vi "Begin.vi"(8 "error in":errorcluster) -> (0 "error out":errorcluster)   [LabVIEW 2014]
doc: "Called before other user functions, this VI is expected to open initial I/O refnums, load in file data, and do all program initialization. Notice that the <B>error out</B> terminal is simply used for data flow. Wiring it to other structures or subVIs ensures that this VI runs first."
uses:
  <vilib>/Rock Robotics/WPI/SafetyOutput/WPI_SafetyOutputConfigMenu.ctl
  <vilib>/Rock Robotics/WPI/DriverStation/WPI_DriverStationRobotMode2.ctl
  <vilib>/Rock Robotics/WPI/Joystick/WPI_JoystickDeviceEnum.ctl
  <vilib>/Rock Robotics/SystemInterfaces/DIO/FPGA_DIOPWMChannel.ctl
  Robot Global Data.vi
  <vilib>/Rock Robotics/Network Tables/SD Write String Array.vi
  <vilib>/Rock Robotics/WPI/RobotDrive/WPI_RobotDriveOpen4MotorWithJaguar.vi
panel:
  in  "error in 2":errorcluster
  out "error out 2":errorcluster
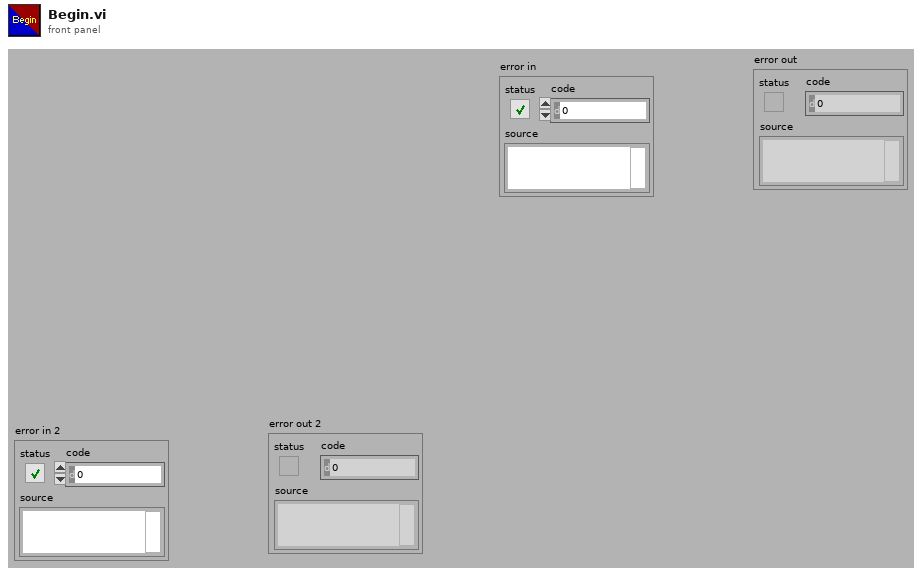
[diagram p1: front panel]
types:
  T1 = typedef "FPGA_DIOPWMChannel.ctl" = enum8{"PWM 0", "PWM 1", "PWM 2", "PWM 3", "PWM 4", "PWM 5", "PWM 6", "PWM 7", "PWM 8", "PWM 9", "PWM MXP 0", "PWM MXP 1", "PWM MXP 2", "PWM MXP 3", "PWM MXP 4", "PWM MXP 5", "PWM MXP 6", "PWM MXP 7", "PWM MXP 8", "PWM MXP 9", "Invalid"}
  T2 = typedef "WPI_JoystickDeviceEnum.ctl" = enum16{"USB 0", "USB 1", "USB 2", "USB 3", "USB 4", "USB 5"}
  T3 = typedef "WPI_DriverStationRobotMode2.ctl" = enum16{"Autonomous Disabled", "Autonomous Enabled", "Teleop Disabled", "Teleop Enabled", "Disconnected", "Finish", "Test Disabled", "Test Enabled", "Emergency Stopped"}
  T4 = typedef "WPI_SafetyOutputConfigMenu.ctl" = enum16{"Enable", "Disable"}
  T5 = typedef "WPI_JoystickDevRef.ctl" = cluster{"Device":T2}
  T6 = typedef "WPI_RobotDriveDevRef.ctl" = cluster{"DevStatus":errorcluster, "Motors[]":T7[], "Square Inputs":bool, "Max Output":dbl}
  T7 = typedef "WPI_MotorControlDeviceRef.ctl" = cluster{"DeviceStatus":errorcluster, "Type":T8, "PWM":cluster{"Controller":T9, "PWM Channel":T1, "DeadBand":T10}, "CAN":cluster{"Device Number":u8, "Control Mode":T11, "Semaphore":T12, "Max Vout":dbl, "TalonSRX Control Mode":T13}, "Invert":bool, "TransformRef":T14, "InvTransformRef":T14}
  T8 = typedef "WPI_MotorControlType.ctl" = enum16{"PWM", "CAN", "CANTalonSRX"}
  T9 = typedef "FPGA_TypedefDigitalModule.ctl" = enum16{"Controller 1"}
  T10 = typedef "WPI_PWMDeadband.ctl" = cluster{"Name":string, "maxPositivePwm":i32, "minPositivePwm":i32, "centerPwm":i32, "maxNegativePwm":i32, "minNegativePwm":i32, "angularRange":u16}
  T11 = typedef "WPI_CANJaguar_ControlMode.ctl" = enum8{"Percent VBus", "Current", "Speed", "Position", "Voltage"}
  T12 = typedef "Semaphore RefNum" = refnum<k1>
  T13 = typedef "WPI_CANTalonSRX_APIControlMode.ctl" = enum8{"Percent VBus", "Speed", "Position", "Slave", "Unchanged / Invalid"}
  T14 = typedef "WPI_PWMTransform_ConPane.ctl" = refnum<vi>
  T15 = typedef "WPI_ServoDeviceRef.ctl" = cluster{"DeviceStatus":errorcluster, "Controller":T9, "PWM Channel":T1, "DeadBand":T10}
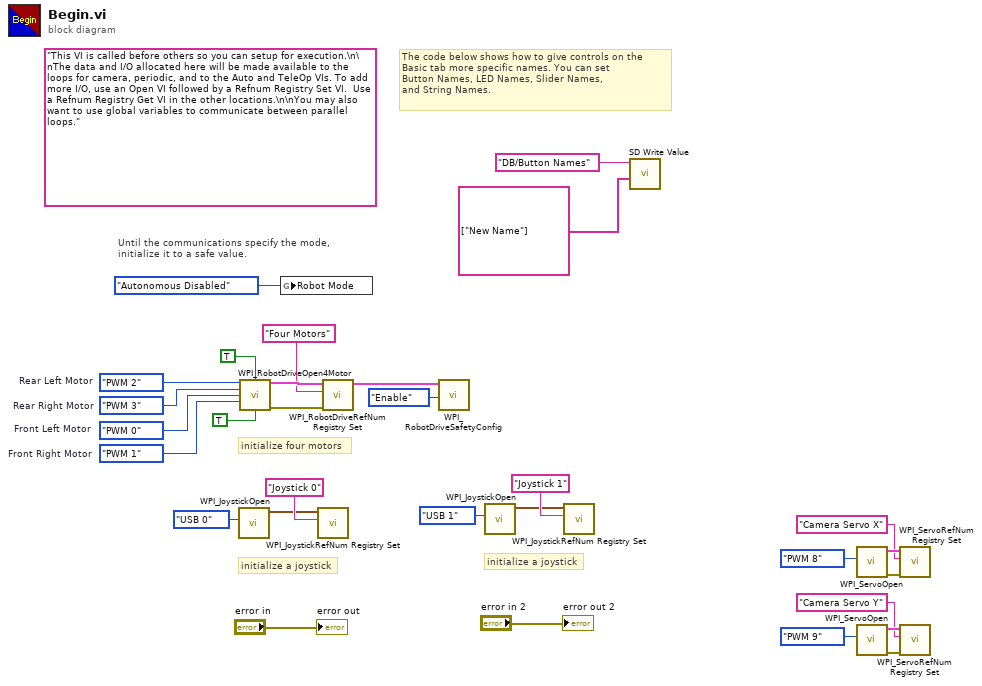
[diagram p0: block diagram]
diagram:
  w18 = FPGA_DIOPWMChannel."PWM 1"  # Front Right Motor
  w19 = FPGA_DIOPWMChannel."PWM 0"  # Front Left Motor
  w20 = FPGA_DIOPWMChannel."PWM 3"  # Rear Right Motor
  w21 = FPGA_DIOPWMChannel."PWM 2"  # Rear Left Motor
  (unwired) "This VI is called before others so you can setup for execution.\n\nThe data and I/O allocated here will be made available to the loops for camera, periodic, and to the Auto and TeleOp VIs. To add more I/O, use an Open VI followed by a Refnum Registry Set VI.  Use a Refnum Registry Get VI in the other locations.\n\nYou may also want to use global variables to communicate between parallel loops."
  # "initialize a joystick"
  # "The code below shows how to give controls on the\nBasic tab more specific names. You can set\nButton Names, LED Names, Slider Names,\nand String Names."
  # "initialize a joystick"
  # "Until the communications specify the mode,\ninitialize it to a safe value."
  # "initialize four motors"
  n1 = call <vilib>:"WPI_JoystickOpen.vi"("JoystickDevice"=WPI_JoystickDeviceEnum."USB 0") -> ("JoystickDevRef"=w23:T5)  [unwired: 10 in]
  n2 = call-poly <vilib>:"WPI_RobotDriveOpen4Motor.vi"("Rear Left Motor"=w21, "Rear Right Motor Inverted"=TRUE, "Rear Right Motor"=w20, "Front Left Motor"=w19, "Front Right Motor"=w18, "Front Right Motor Inverted"=TRUE) -> ("RobotDriveDevRef"=w30:T6, "error out"=w28:errorcluster)  [unwired: 8 in]
  n3 = global write "Robot Global Data.vi" "Robot Mode"(WPI_DriverStationRobotMode2."Autonomous Disabled" ("Robot Mode")) -> ()
  n4 = call <vilib>:"WPI_JoystickRefNum Registry Set.vi"("refnum name"="Joystick 0", "JoystickDevRef"=w23) -> ()  [unwired: 8 in, 2 out]
  n5 = call <vilib>:"WPI_RobotDriveRefNum Registry Set.vi"("error in (no error)"=w28, "refnum name"="Four Motors", "RobotDriveDevRef"=w30) -> ("RobotDriveDevRef"=w27:T6)  [unwired: 8 out]
  n6 = call <vilib>:"WPI_RobotDriveSafetyConfig.vi"("mode"=WPI_SafetyOutputConfigMenu."Enable", "RobotDriveDevRef"=w27) -> ()  [unwired: 8 in, 2 out]
  n7 = call <vilib>:"WPI_JoystickOpen.vi"("JoystickDevice"=WPI_JoystickDeviceEnum."USB 1") -> ("JoystickDevRef"=w13:T5)  [unwired: 10 in]
  n8 = call <vilib>:"WPI_JoystickRefNum Registry Set.vi"("refnum name"="Joystick 1", "JoystickDevRef"=w13) -> ()  [unwired: 8 in, 2 out]
  n9 = call-poly <vilib>:"SD Write Value.vi"("String Array"=string[] ["New Name"], "Name"="DB/Button Names") -> ()  [unwired: 8 in, 2 out]
  n10 = call <vilib>:"WPI_ServoOpen.vi"("PWM Channel"=FPGA_DIOPWMChannel."PWM 8") -> ("error out"=w7:errorcluster, "ServoDeviceRef"=w8:T15)  [unwired: 9 in]
  n11 = call <vilib>:"WPI_ServoOpen.vi"("PWM Channel"=FPGA_DIOPWMChannel."PWM 9") -> ("error out"=w4:errorcluster, "ServoDeviceRef"=w5:T15)  [unwired: 9 in]
  n12 = call <vilib>:"WPI_ServoRefNum Registry Set.vi"("error in (no error)"=w7, "refnum name"="Camera Servo X", "ServoDeviceRef"=w8) -> ()  [unwired: 7 in, 2 out]
  n13 = call <vilib>:"WPI_ServoRefNum Registry Set.vi"("error in (no error)"=w4, "refnum name"="Camera Servo Y", "ServoDeviceRef"=w5) -> ()  [unwired: 7 in, 2 out]
  "error out" <- "error in"
  "error out 2" <- "error in 2"
